vi "GOOP_LVClass_Global_Init.vi"(11 "Object":u64) -> ()   [LabVIEW 2020]
doc: "NI Confidential \n\n/**\n@brief This VI is called by the framework when an item of this type is first created.\n\n@author Joel Dixon\n\n@par Sample_Item_Init.vi\n This VI might typically set the popup menu for this item by calling mxLvSetPopupMenu.vi, set the icon for the item by calling mxLvSetIcon.vi, and set a name to be displayed in the tree by calling mxLvSetName.vi. \n\n@param \"Object\" [in] \nPassed by the framework as a reference to 'this' item in the tree. This parameter can be passed as the 'item' parameter for any of the mxLv** VIs, such as mxLvCreateItems.vi.\n*/"
uses:
  <resource>/Framework/Providers/API/mxLvMenuItem.ctl
  <resource>/Framework/Providers/Open_GDS/ClassProviders/Provider_EndevoGOOP300/ClassWriterGOOP300_class/ClassWriterGOOP300.lvclass
  <resource>/Framework/Providers/Open_GDS/ClassProviders/Provider_LvNativeClass/ClassWriterNative_class/ClassWriterNative.lvclass
  <resource>/Framework/Providers/Open_GDS/ClassProviders/Provider_EndevoGOOP300/ClassReaderGOOP300_class/ClassReaderGOOP300.lvclass
  <resource>/Framework/Providers/Open_GDS/ClassProviders/Provider_LvNativeClass/ClassReaderNative_class/ClassReaderNative.lvclass
  <resource>/Framework/Providers/Open_GDS/ClassProviders/Provider_EndevoGOOP400/ClassWriterGOOP400_class/ClassWriterGOOP400.lvclass
  <resource>/Framework/Providers/Open_GDS/ClassProviders/Provider_EndevoGOOP400/ClassReaderGOOP400_class/ClassReaderGOOP400.lvclass
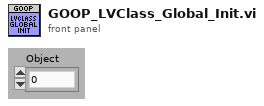
[diagram p1: front panel]
types:
  T1 = typedef "mxLvMenuItem.ctl" = cluster{"Menu Name":string, "Description":string, "Icon File Name":path, "Menu Tag":string, "Enabled":bool, "Checked":bool, "Separator":bool, "Batchable":bool, "Weight":i32, "Batch Mode (Ignored if Not Batchable)":enum32{"Show If All Items Support Command", "Show If Any Items Support Command"}, "Menu Location":enum32{"<None>", "Project", "Project / Build Specifications", "Tools", "Tools / Source Control", "Tools / Real-Time Module", "Help"}, "Exclude From Getting Started Window Menu":bool}
  T2 = typedef "GdsLanguage_LanguageID.ctl" = enum16{"< undefined >", "aa", "ab", "af", "am", "ar", "as", "ay", "az", "ba", "be", "bg", "bh", "bi", "bn", "bo", "br", "ca", "co", "cs", "cy", "da", "de", "dz", "el", "en", "eo", "es", "et", "eu", "fa", "fi", "fj", "fo", "fr", "fy", "ga", "gd", "gl", "gn", "gu", "gv", "ha", "he", "hi", "hr", "hu", "hy", "ia", "id", "ie", "ik", "is", "it", "iu", "ja", "jv", "ka", "kk", "kl", "km", "kn", "ko", "ks", "ku", "ky", "la", "li", "ln", "lo", "lt", "lv", "mg", "mi", "mk", "ml", "mn", "mo", "mr", "ms", "mt", "my", "na", "ne", "nl", "no", "oc", "om", "or", "pa", "pl", "ps", "pt", "qu", "rm", "rn", "ro", "ru", "rw", "sa", "sd", "sg", "sh", "si", "sk", "sl", "sm", "sn", "so", "sq", "sr", "ss", "st", "su", "sv", "sw", "ta", "te", "tg", "th", "ti", "tk", "tl", "tn", "to", "tr", "ts", "tt", "tw", "ug", "uk", "ur", "uz", "vi", "vo", "wo", "xh", "yi", "yo", "zh", "zu"}
  T3 = enum32{"Bad", "Idle", "Run top level", "Running"}
  T4 = typedef "ItemRef.ctl" = u64
  T5 = enum32{"invalid OS target", "Mac OS", "Windows 3.1", "Windows 95/NT", "Solaris 1", "Solaris 2", "HP-UX", "PowerMAX", "Linux", "Irix", "Rhapsody", "BeOS", "AIX", "OSF1", "VxWorks", "PharLap", "Carbon", "RTX", "Windows x64", "Linux x64"}
  T6 = enum32{"invalid OS target", "Mac OS", "Windows 3.1", "Windows 95/NT", "Solaris 1", "Solaris 2", "HP-UX", "PowerMAX", "Linux", "Irix", "Rhapsody", "BeOS", "AIX", "OSF1", "VxWorks", "PharLap", "Carbon", "RTX", "Windows x64", "Linux x64", "Mac OS X x64"}
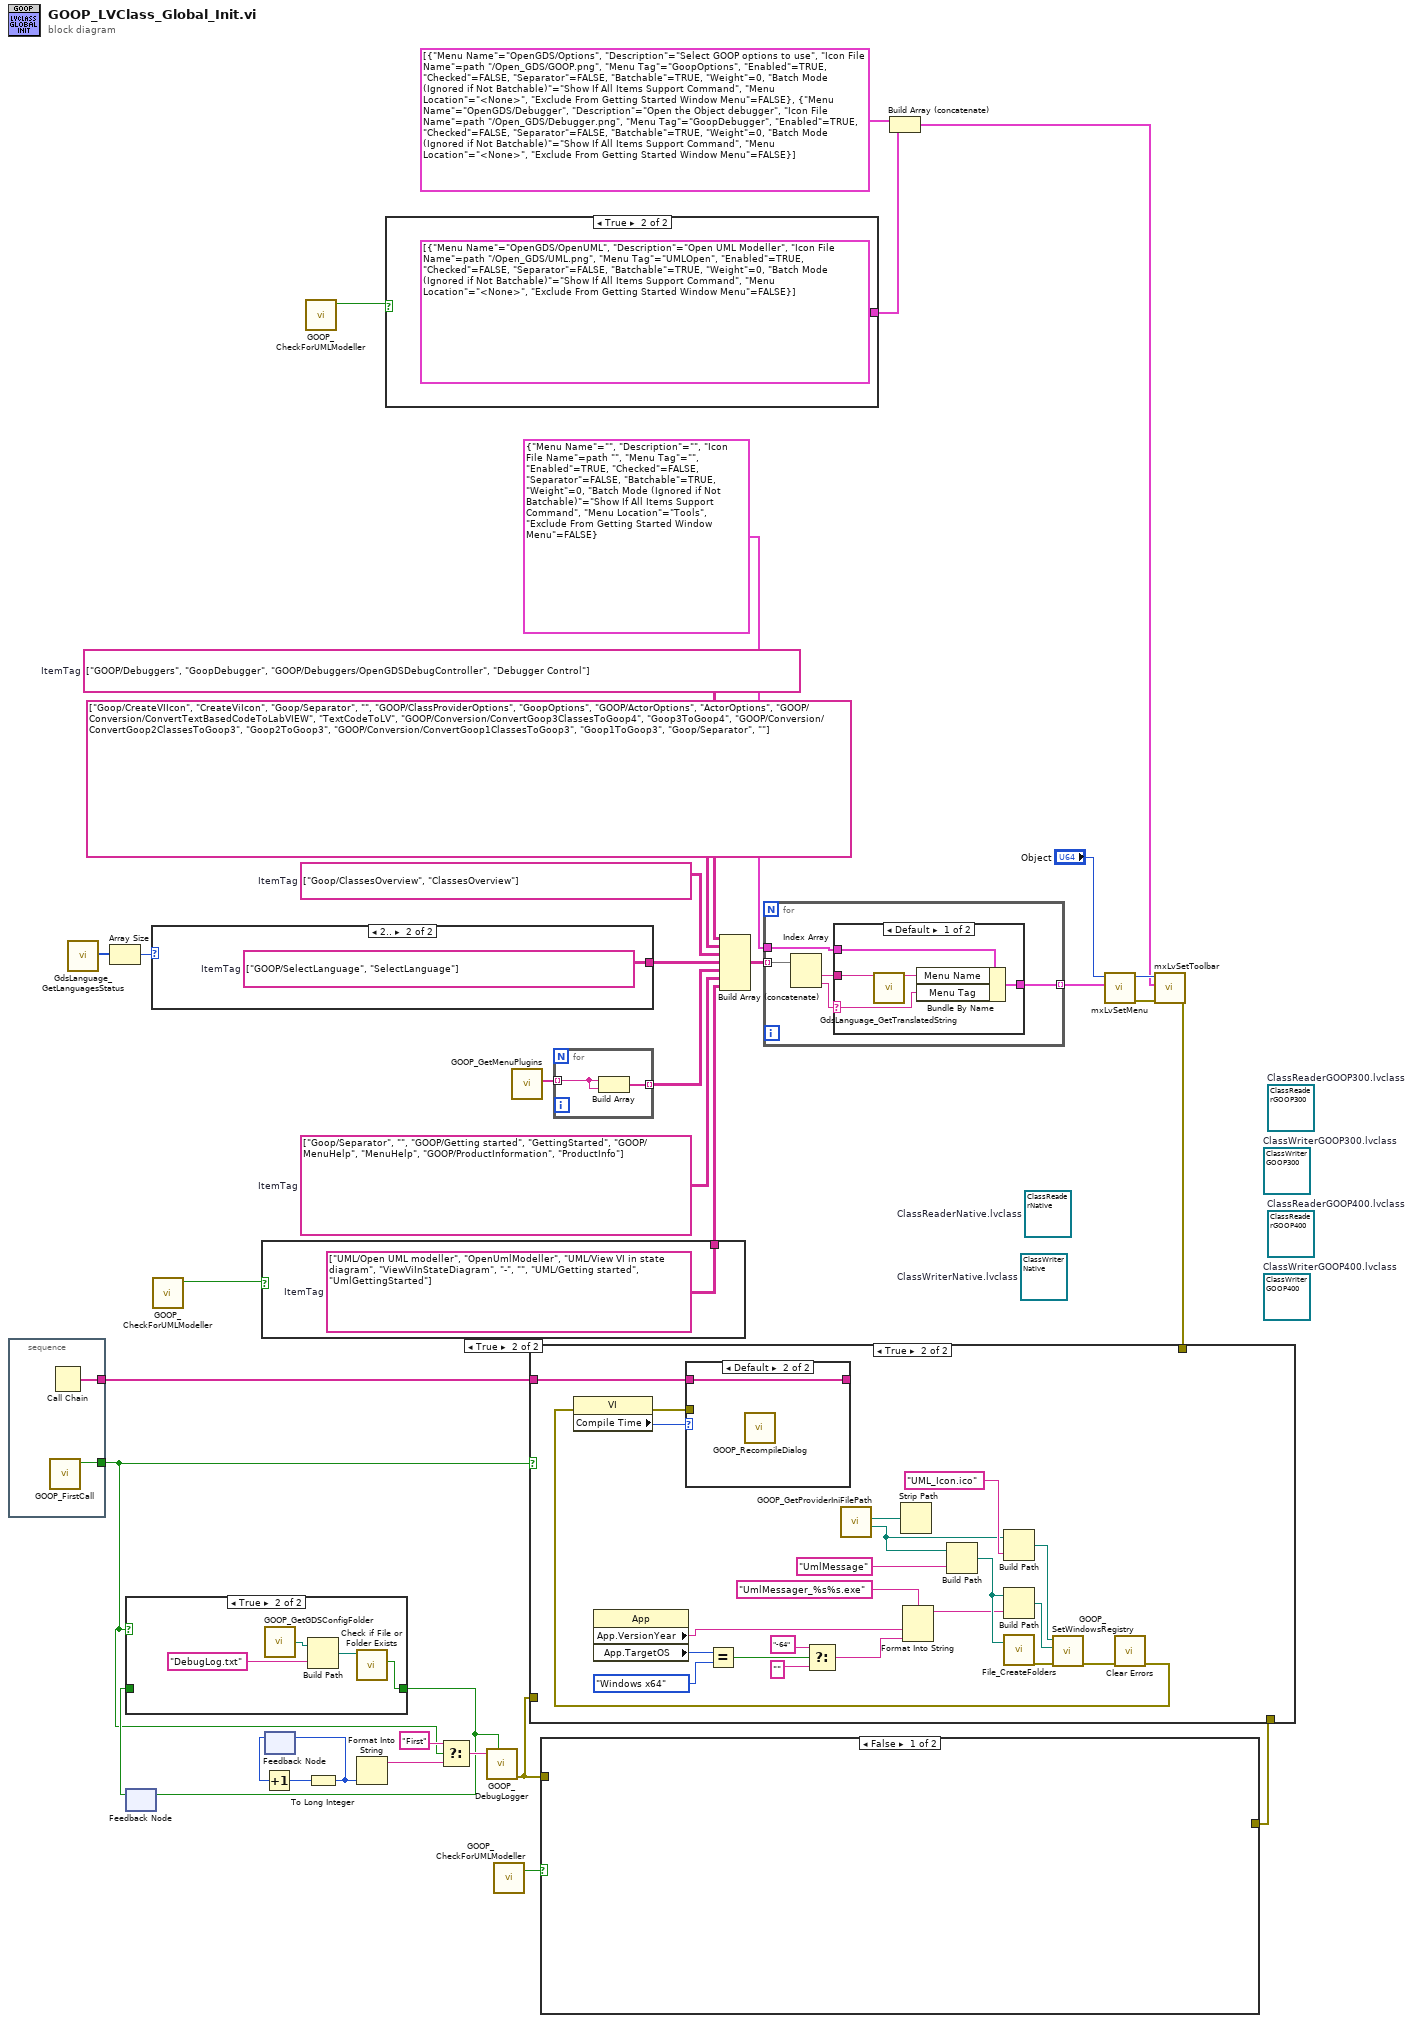
[diagram p0: block diagram]
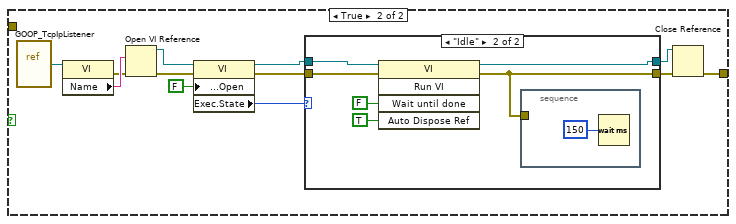
[diagram p4: hidden frame]
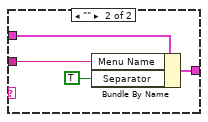
[diagram p6: hidden frame]
diagram:
  w11 = string[][] [["Goop/ClassesOverview", "ClassesOverview"]]  # ItemTag
  w23 = string[][] [["GOOP/Debuggers", "GoopDebugger"], ["GOOP/Debuggers/OpenGDSDebugController", "Debugger Control"]]  # ItemTag
  (unwired) refnum<class "ClassReaderGOOP400.lvclass"> refnum  # ClassReaderGOOP400.lvclass
  (unwired) refnum<class "ClassWriterGOOP400.lvclass"> refnum  # ClassWriterGOOP400.lvclass
  (unwired) refnum<class "ClassReaderNative.lvclass"> refnum  # ClassReaderNative.lvclass
  (unwired) refnum<class "ClassReaderGOOP300.lvclass"> refnum  # ClassReaderGOOP300.lvclass
  (unwired) refnum<class "ClassWriterNative.lvclass"> refnum  # ClassWriterNative.lvclass
  (unwired) refnum<class "ClassWriterGOOP300.lvclass"> refnum  # ClassWriterGOOP300.lvclass
  w15 = string[][] [["Goop/Separator", ""], ["GOOP/Getting started", "GettingStarted"], ["GOOP/MenuHelp", "MenuHelp"], ["GOOP/ProductInformation", "ProductInfo"]]  # ItemTag
  n1 = stacked-sequence {
    tunnel: [w37] -> w28
    tunnel: [w36] -> w9
    frame #0 {
      n2 = call <resource>:"GOOP_FirstCall.vi"() -> ("First Call?: T/F"=w37:bool)  [unwired: 11 in]
      n3 = Call Chain() -> (call chain=w36:string[])
    }
  }
  n4 = call <resource>:"GdsLanguage_GetLanguagesStatus.vi"() -> ("FoundLanguages"=w26:T2[])  [unwired: 16 in, 3 out]
  n5 = Array Size(array=w26) -> (size(s)=w21:i32)
  n6 = feedback #1() -> (w29:bool)  [unwired: 1 in]
  n7 = case shown="True" w28 {
    tunnel: [w38 w40] -> w27
    tunnel: w29 -> [w38 _]
    frame False {
    }
    frame True {
      n8 = call <resource>:"GOOP_GetGDSConfigFolder.vi"() -> ("GDSFolderPath"=w39:path)
      n9 = Build Path(base path=w39, name or relative path="DebugLog.txt") -> (appended path=w42:path)
      n10 = call <vilib>:"Check if File or Folder Exists.vi"("path"=w42) -> ("file or folder exists?"=w40:bool)  [unwired: 8 in, 2 out]
    }
  }
  n11 = feedback-in #1(w27) -> ()
  n12 = case shown="2.." w21 {
    tunnel: [_ w43] -> w16
    frame Default {
    }
    frame 2.. {
      w43 = string[][] [["GOOP/SelectLanguage", "SelectLanguage"]]  # ItemTag
    }
  }
  n13 = call <resource>:"GOOP_CheckForUMLModeller.vi"() -> ("UML Modeller Exists"=w4:bool)  [unwired: 10 in, 1 out]
  n14 = case shown="True" w4 {
    tunnel: [_ w44] -> w14
    frame False {
    }
    frame True {
      w44 = string[][] [["UML/Open UML modeller", "OpenUmlModeller"], ["UML/View VI in state diagram", "ViewViInStateDiagram"], ["-", ""], ["UML/Getting started", "UmlGettingStarted"]]  # ItemTag
    }
  }
  n15 = feedback #2() -> (w33:i32)  [unwired: 1 in]
  n16 = Increment(x=w33) -> (x+1=w32:i32)
  n17 = call <resource>:"GOOP_CheckForUMLModeller.vi"() -> ("UML Modeller Exists"=w1:bool)  [unwired: 10 in, 1 out]
  n18 = To Long Integer(number=w32) -> (32bit integer=w31:i32)
  n19 = feedback-in #2(w31) -> ()
  n20 = Format Into String(w31) -> (resulting string=w30:string)  [unwired: 3 in, 1 out]
  n21 = case shown="True" w1 {
    tunnel: [_ T1[] [{"Menu Name"="OpenGDS/OpenUML", "Description"="Open UML Modeller", "Icon File Name"=path "../Open_GDS/UML.png", "Menu Tag"="UMLOpen", "Enabled"=TRUE, "Checked"=FALSE, "Separator"=FALSE, "Batchable"=TRUE, "Weight"=0, "Batch Mode (Ignored if Not Batchable)"=enum."Show If All Items Support Command", "Menu Location"=enum."<None>", "Exclude From Getting Started Window Menu"=FALSE}] ("Menu Items")] -> w2
    frame False {
    }
    frame True {
    }
  }
  n22 = Select(t="First" ("name or relative path"), s=w28, f=w30) -> (s? t:f=w35:string)
  n23 = call <resource>:"GOOP_DebugLogger.vi"("ActivateDebugging"=w27, "State"=w35) -> ("error out"=w5:errorcluster)  [unwired: 7 in, 2 out]
  n24 = call <resource>:"GOOP_CheckForUMLModeller.vi"() -> ("UML Modeller Exists"=w6:bool)  [unwired: 10 in, 1 out]
  n25 = call <resource>:"GOOP_GetMenuPlugins.vi"() -> ("MenuPlugins(E.g. GOOP/My function)"=w13:string[])  [unwired: 10 in, 1 out]
  n26 = case shown="False" w6 {
    tunnel: [_ w57] -> w8
    tunnel: w5 -> [_ _]
    frame False {
    }
    frame True {
      n27 = vi-ref <resource>:"GOOP_TcpIpListener.vi"() -> (w56:refnum<vi>)
      n28 = property class="VI"(reference=w56) -> (error out=w54:errorcluster, "Name"=w55:string)  [unwired: 1 in, 1 out]
      n29 = Open VI Reference(vi path=w55, error in (no error)=w54) -> (vi reference=w53:refnum<vi>, error out=w52:errorcluster)  [unwired: 4 in]
      n30 = property class="VI"(reference=w53, error in=w52, "Front Panel.Open"=FALSE ("Front Panel Window:Open")) -> (reference out=w50:refnum<vi>, error out=w49:errorcluster, "Exec.State"=w48:T3)
      n31 = case shown="\"Idle\"" w48 {
        tunnel: [w59 w63] -> w47
        tunnel: w50 -> [w59 w62]
        tunnel: w49 -> [w58 w61]
        tunnel: [w58 w60] -> w46
        frame "Bad", Default {
        }
        frame "Idle" {
          n32 = invoke class="VI" method="Run VI"(reference=w62, error in=w61, "Wait until done"=FALSE ("Wait Until Done"), "Auto Dispose Ref"=TRUE ("Wait Until Done")) -> (reference out=w63:refnum<vi>, error out=w60:errorcluster)  [unwired: 1 in, 3 out]
          n33 = stacked-sequence {
            tunnel: w60 -> [_]
            frame #0 {
              n34 = Wait (ms)(milliseconds to wait=u32 150) -> ()  [unwired: 1 out]
            }
          }
        }
      }
      n35 = Close Reference(reference=w47, error in (no error)=w46) -> (error out=w57:errorcluster)
    }
  }
  n36 = for {
    tunnel: w13 -> [w68] mode=indexing
    tunnel: [w67] -> w12 mode=indexing
    n37 = Build Array(w68, w68) -> (w67:string[])
  }
  n38 = Build Array (concatenate)(w23, string[][] [["Goop/CreateVIIcon", "CreateViIcon"], ["Goop/Separator", ""], ["GOOP/ClassProviderOptions", "GoopOptions"], ["GOOP/ActorOptions", "ActorOptions"], ["GOOP/Conversion/ConvertTextBasedCodeToLabVIEW", "TextCodeToLV"], ["GOOP/Conversion/ConvertGoop3ClassesToGoop4", "Goop3ToGoop4"], ["GOOP/Conversion/ConvertGoop2ClassesToGoop3", "Goop2ToGoop3"], ["GOOP/Conversion/ConvertGoop1ClassesToGoop3", "Goop1ToGoop3"], ["Goop/Separator", ""]] ("ItemTag"), w11, w16, w12, w15, w14) -> (w20:string[][])
  n39 = for {
    tunnel: w20 -> [w73] mode=indexing
    tunnel: T1 {"Menu Name"="", "Description"="", "Icon File Name"=path "", "Menu Tag"="", "Enabled"=TRUE, "Checked"=FALSE, "Separator"=FALSE, "Batchable"=TRUE, "Weight"=0, "Batch Mode (Ignored if Not Batchable)"=enum."Show If All Items Support Command", "Menu Location"=enum."Tools", "Exclude From Getting Started Window Menu"=FALSE} ("Menu Item") -> [w72]
    tunnel: [w69] -> w18 mode=indexing
    n40 = Index Array(array=w73) -> (element #1=w70:string, element #2=w71:string)  [unwired: 2 in]
    n41 = case shown="Default" w71 {
      selector: w71 -> [w75 _]
      tunnel: w72 -> [w78 w80]
      tunnel: w70 -> [w76 w82]
      tunnel: [w74 w79] -> w69
      frame Default {
        n42 = call <resource>:"GdsLanguage_GetTranslatedString.vi"("StringID(s)"=w76) -> ("FirstStringOut"=w77:string)  [unwired: 15 in, 3 out]
        n43 = Bundle By Name(cluster=w78, "Menu Name"=w77, "Menu Tag"=w75) -> (w74:T1)
      }
      frame "" {
        n44 = Bundle By Name(cluster=w80, "Menu Name"=w82, "Separator"=TRUE) -> (w79:T1)
      }
    }
  }
  n45 = Build Array (concatenate)(T1[] [{"Menu Name"="OpenGDS/Options", "Description"="Select GOOP options to use", "Icon File Name"=path "../Open_GDS/GOOP.png", "Menu Tag"="GoopOptions", "Enabled"=TRUE, "Checked"=FALSE, "Separator"=FALSE, "Batchable"=TRUE, "Weight"=0, "Batch Mode (Ignored if Not Batchable)"=enum."Show If All Items Support Command", "Menu Location"=enum."<None>", "Exclude From Getting Started Window Menu"=FALSE}, {"Menu Name"="OpenGDS/Debugger", "Description"="Open the Object debugger", "Icon File Name"=path "../Open_GDS/Debugger.png", "Menu Tag"="GoopDebugger", "Enabled"=TRUE, "Checked"=FALSE, "Separator"=FALSE, "Batchable"=TRUE, "Weight"=0, "Batch Mode (Ignored if Not Batchable)"=enum."Show If All Items Support Command", "Menu Location"=enum."<None>", "Exclude From Getting Started Window Menu"=FALSE}] ("Menu Items"), w2) -> (w3:T1[])
  n46 = call <resource>:"mxLvSetMenu.vi"("Menu Items"=w18, "Item"="Object") -> ("error out"=w17:errorcluster, "Item"=w25:T4)  [unwired: 8 in]
  n47 = call <resource>:"mxLvSetToolbar.vi"("error in"=w17, "Toolbar Items"=w3, "Item"=w25) -> ("error out"=w7:errorcluster)  [unwired: 7 in, 1 out]
  n48 = case shown="True" w28 {
    tunnel: w5 -> [_ _]
    tunnel: w9 -> [_ w86]
    tunnel: w8 -> [_ _]
    tunnel: w7 -> [_ _]
    frame False {
    }
    frame True {
      n49 = property class="App"() -> ("App.VersionYear"=w102:string, "App.TargetOS"=w94:T6)  [unwired: 2 in, 2 out]
      n50 = Equal?(x=w94, y=T5."Windows x64") -> (x = y?=w93:bool)
      n51 = Select(t="-64" ("string"), s=w93, f="" ("string")) -> (s? t:f=w92:string)
      n52 = call <resource>:"GOOP_GetProviderIniFilePath.vi"() -> ("ProviderMainFolder"=w83:path, "ProviderIniPath"=w89:path)  [unwired: 10 in]
      n53 = Strip Path(path=w89) -> ()  [unwired: 2 out]
      n54 = Format Into String(format string="UmlMessager_%s%s.exe", w102, w92) -> (resulting string=w100:string)  [unwired: 2 in, 1 out]
      n55 = Build Path(base path=w83, name or relative path="UmlMessage") -> (appended path=w101:path)
      n56 = Build Path(base path=w83, name or relative path="UML_Icon.ico") -> (appended path=w97:path)
      n57 = Build Path(base path=w101, name or relative path=w100) -> (appended path=w99:path)
      n58 = call <resource>:"File_CreateFolders.vi"("Path"=w101) -> ("error out"=w96:errorcluster)  [unwired: 16 in, 2 out]
      n59 = call <resource>:"GOOP_SetWindowsRegistry.vi"("error in (no error)"=w96, "ExeFile"=w99, "IconFile"=w97) -> ("error out"=w85:errorcluster)  [unwired: 8 in]
      n60 = call <vilib>:"Clear Errors.vi"("error in (no error)"=w85) -> ("error out"=w84:errorcluster)  [unwired: 5 in, 1 out]
      n61 = property class="VI"(error in=w84) -> (error out=w87:errorcluster, "Compile Time"=w88:i32)  [unwired: 1 in, 1 out]
      n62 = case shown="Default" w88 {
        tunnel: w87 -> [_ _]
        tunnel: w86 -> [_ w105]
        tunnel: [_ w105] -> _
        frame 0 {
        }
        frame Default {
          n63 = call <resource>:"GOOP_RecompileDialog.vi"() -> ()  [unwired: 19 in, 1 out]
        }
      }
    }
  }
